vi "main_tweezer_program.vi"() -> ()   [LabVIEW 2017]
uses:
  <vilib>/userdefined/High Color/IMAQdx.ctl
  Serial - Settings.ctl
  <vilib>/Platform/TimedLoop/XDataNode/timing_clust.ctl
  <vilib>/Platform/TimedLoop/XDataNode/nitl_modes.ctl
  <vilib>/Platform/TimedLoop/XDataNode/wakeup.ctl
  C:/Users/mcroning/Documents/builds/Tweezers211_2020/Optical Tweezers Source Tufts/ThorLabs.MotionControl.KCube.PositionAlignerCLI.dll
  ThorLabs.MotionControl.KCube.PositionAlignerCLI.dll
  <vilib>/DAQmx/read.llb/DAQmx Read (Analog DBL 1Chan 1Samp).vi
  <vilib>/DAQmx/write.llb/DAQmx Write (Analog DBL 1Chan 1Samp).vi
  <vilib>/DAQmx/write.llb/DAQmx Write (Analog 1D DBL NChan 1Samp).vi
  <vilib>/DAQmx/read.llb/DAQmx Read (Analog 1D DBL NChan 1Samp).vi
  <vilib>/Analysis/baseanly.llb/Mean (DBL).vi
  <extravilib>/ChannelInstances/Tag-bool/Read With Abort.vi
  <extravilib>/ChannelInstances/Tag-bool/Write With Abort.vi
  <vilib>/DAQmx/create/channels.llb/DAQmx Create Channel (AI-Voltage-Basic).vi
  <vilib>/DAQmx/create/channels.llb/DAQmx Create Channel (AO-Voltage-Basic).vi
  <vilib>/Instr/_visa.llb/VISA Configure Serial Port (Instr).vi
  <vilib>/DAQmx/miscellaneous.llb/DAQmx Fill In Error Info.vi
  <vilib>/Utility/inputDevices.llb/mouseAcquire.vi
  <extravilib>/ChannelInstances/Tag-bool/Instantiate.vi
  <extravilib>/ChannelInstances/Tag-bool/EndpointRead.vi
  <extravilib>/ChannelInstances/Tag-bool/Endpoint.vi
  <vilib>/addons/control/pid/pid.llb/PID (DBL).vi
  <vilib>/platform/TimedLoop/XDataNode/XDataNode.xnode
  <vilib>/vision/driver/NI_Vision_Acquisition_Software.lvlib
  C:/Users/mcroning/Documents/builds/Tweezers211_2020/Optical Tweezers Source Tufts/Thorlabs.MotionControl.Controls.dll
  Thorlabs.MotionControl.Controls.dll
  <extravilib>/ChannelInstances/Tag-bool.lvlib
  <vilib>/addons/control/pid/NI_PID_autopid.lvlib
  <vilib>/Platform/TimedLoop/XDataNode/XDNodeRunTimeDep.lvlib
  <vilib>/Analysis/NI_AALBase.lvlib
  <vilib>/addons/control/pid/NI_PID_pid.lvlib
  C:/Program Files (x86)/National Instruments/LabVIEW 2017/resource/objmgr/imaqdx.rc
panel:
  in  "Period":i64
  out "Mean Temp":dbl
  out "Mean magnitude":dbl
  out "Mean phase":dbl
  in  "Tab Control":T1(tab)
  in  "Exposure time LS":i32=25000
  in  "Frame rate LS":i32=30
  out "Sensor Readout Mode":string
  in  "Number of Images":i32=5
  in  "Exposure time LSwhile run":i32=30000
  out "Bead":cluster{"X":dbl, "Y":dbl}
  out "Score":i32
  in  "Learn Bead for Tracking":bool
  out "Bead Learned":bool
  in  "autotuning parameters":T2={"controller type"=1, "relay cycles"=3, "relay amplitude"=1.0, "control specification"=2, "PV noise level"=0.1} {"PV noise level" format="%.2f"; "control specification" items=["normal", "fast", "slow"]; "relay amplitude" format="%.2f"; "controller type" items=["PID", "PI", "P"]}
  in  "PID gains":T3={"proportional gain (Kc)"=0.398, "integral time (Ti, min)"=0.01577, "derivative time (Td, min)"=0.0} {"derivative time (Td, min)" format="%.3f"; "integral time (Ti, min)" format="%.3f"; "proportional gain (Kc)" format="%.3f"}
  out "Autotuning PID gains out":T3={"proportional gain (Kc)"=1.0, "integral time (Ti, min)"=0.01, "derivative time (Td, min)"=0.0} {"derivative time (Td, min)" format="%.3f"; "integral time (Ti, min)" format="%.3f"; "proportional gain (Kc)" format="%.3f"}
  out "Heater voltage":dbl format="%.2f"
  in  "Temperature \nupdate period ms":i64=10
  in  "autotune? (F)":bool
  in  "Switch control xy":bool=TRUE
  out "output top":dbl format="%.2e"
  in  "top g pos":bool=TRUE
  in  "bottom g pos":bool=TRUE
  in  "PID pos lock":T3={"proportional gain (Kc)"=1.0, "integral time (Ti, min)"=0.01, "derivative time (Td, min)"=0.0} {"derivative time (Td, min)" format="%.3f"; "integral time (Ti, min)" format="%.3f"; "proportional gain (Kc)" format="%.3f"}
  out "Acum nudge x":dbl
  out "Acum nudge y":dbl
  in  "nudge x+":bool
  in  "nudge y+":bool
  in  "nudge x-":bool
  in  "nudge y-":bool
  in  "Nudge x":dbl min=-0.1 max=0.1 step=0.0001
  in  "Nudge y":dbl min=-0.1 max=0.1 step=0.0001
  out "lock in range x":bool
  out "lock in range y":bool
  out "|X Steering Voltage|<1":bool
  out "|Y Steering Voltage|<1":bool
  in  "proportional":dbl=1.0
  in  "integral":dbl
  in  "differential":dbl
  in  "update PID":bool
  out "Sum":dbl
  out "X demand position":dbl
  out "Y demand position":dbl
  out "lock in range x 2":bool
  out "lock in range y 2":bool
  in  "demand signal scale":dbl=0.1
  out "data to write":dbl[][](array[numeric])
  in  "Record Data":bool
  in  "Write to  file":bool
  out "steering voltages":dbl[](array[numeric])
  in  "lock on":bool
  in  "Set Frequency":dbl=1.0
  out "Objective monitor":dbl
  out "Phase":dbl
  out "ResponseMagnitude":dbl
  out "Temp C":dbl
  in  "Temp Setpoint":dbl format="%.2f"
  out "clicks":i32
  out "Image 2":T4(plugin-control)
  in  "stop":bool
  in  "KCubePositionAlignerControl 2":refnum<k24>(container)
  out "Mouse Initialized":bool
  out "Calib pt":i32
  in  "Calibrate Mouse":bool
  in  "Calib scale":dbl=0.1
  in  "Mouse Active":bool
  out "Y":dbl
  out "X":dbl
  in  "Focus Increment":dbl=0.1 min=0.0 max=1.0 step=0.001
  in  "Focus out":dbl min=0.0 max=10.0 step=0.01
  # "Program designed for automatic rheology measurements"
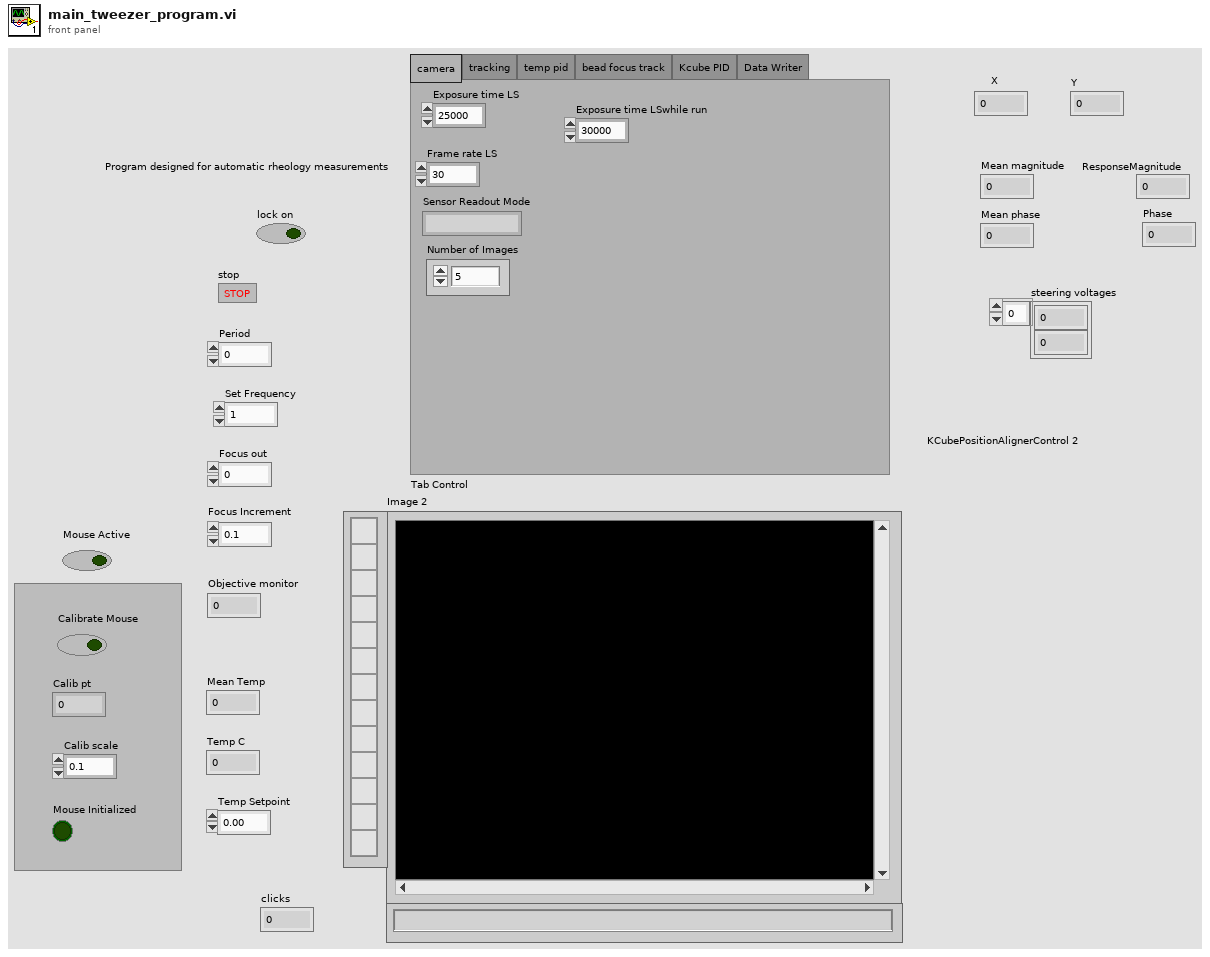
[diagram p1: front panel]
types:
  T1 = enum32{"camera", "tracking", "temp pid", "bead focus track", "Kcube PID", "Data Writer"}
  T2 = cluster{"controller type":u16, "relay cycles":i32, "relay amplitude":dbl, "control specification":u16, "PV noise level":dbl}
  T3 = cluster{"proportional gain (Kc)":dbl, "integral time (Ti, min)":dbl, "derivative time (Td, min)":dbl}
  T4 = typedef "IMAQ Image.ctl" = refnum<image>
  T5 = typedef "Serial - Settings.ctl" = cluster{"baud rate":u32, "data bits":u16, "parity":enum16{"None", "Odd", "Even", "Mark", "Space"}, "stop bits":u16, "flow control":u16}
  T6 = typedef "IMAQdx.ctl" = refnum<k21>
  T7 = typedef "IMAQ Object Tracking Session.ctl" = refnum<k20>
  T8 = cluster{cluster{"Horizontal":i32, "Vertical":i32}, dbl[]}[]
  T9 = cluster{"button 1":bool, "button 2":bool, "button 3":bool, "button 4":bool}
  T10 = cluster{"Horizontal":i32, "Vertical":i32, "Scrolling":i32}
  T11 = cluster{cluster{"Horizontal":i32, "Vertical":i32}, dbl[]}
  T12 = typedef "NI_Matrix.lvlib/RealMatrix.ctl" = dbl[][]
  T13 = cluster{"transformation matrix":T12, "offset":dbl[]}
  T14 = typedef "LVPoint32TypeDef.ctl" = cluster{"Horizontal":i32, "Vertical":i32}
  T15 = cluster{"Global Rectangle":i32[], "Contours":cluster{"Contour Type":u32, "ROI Type":u32, "Points":i32[]}[]}
  T16 = typedef "XDNodeRunTimeDep.lvlib/timing_clust.ctl" = cluster{"Expected End [f-1]":u64, "Actual End [f-1]":u64, "Finished Late? [f-1]":bool, "Expected End [i-1]":u64, "Actual End [i-1]":u64, "Finished Late? [i-1]":bool, "Expected Start [i]":u64, "Actual Start [i]":u64, "Expected Start [f]":u64, "Actual Start [f]":u64, "Source Name":string, "Structure Name":string, "Period":i64, "Deadline":i64, "Offset":i64, "Start":i64, "Priority":i32, "Timeout":i32, "Mode":T17, "Wakeup Reason":T18, "Error":errorcluster, "Source Type":string, "Secondary Source Type":string, "Global End Time":u64, "Global Start Time":u64, "Frame Duration":u64, "Iteration Duration":u64, "Assigned CPU":i32, "I/O Scan Engine Mode":u32}
  T17 = typedef "XDNodeRunTimeDep.lvlib/nitl_modes.ctl" = enum32{"No Change", "Process missed periods, maintain original phase", "Discard missed periods, maintain original phase", "Process missed periods, ignore original phase", "Discard missed periods, ignore original phase"}
  T18 = typedef "XDNodeRunTimeDep.lvlib/wakeup.ctl" = enum32{"Normal", "Aborted", "Asynchronous wakeup", "Timing source error", "Timed loop error", "Timeout"}
  T19 = cluster{"Label":string, "Score":i32, "Angle":dbl, "Location":cluster{"X":dbl, "Y":dbl}, "Bounding Box":cluster{"X":dbl, "Y":dbl}[], "Object Found?":bool}[]
  T20 = cluster{"Label":string, "Score":i32, "Angle":dbl, "Location":cluster{"X":dbl, "Y":dbl}, "Bounding Box":cluster{"X":dbl, "Y":dbl}[], "Object Found?":bool}
  T21 = typedef "Tag-bool.lvlib/))Channel.ctl" = refnum<queue>
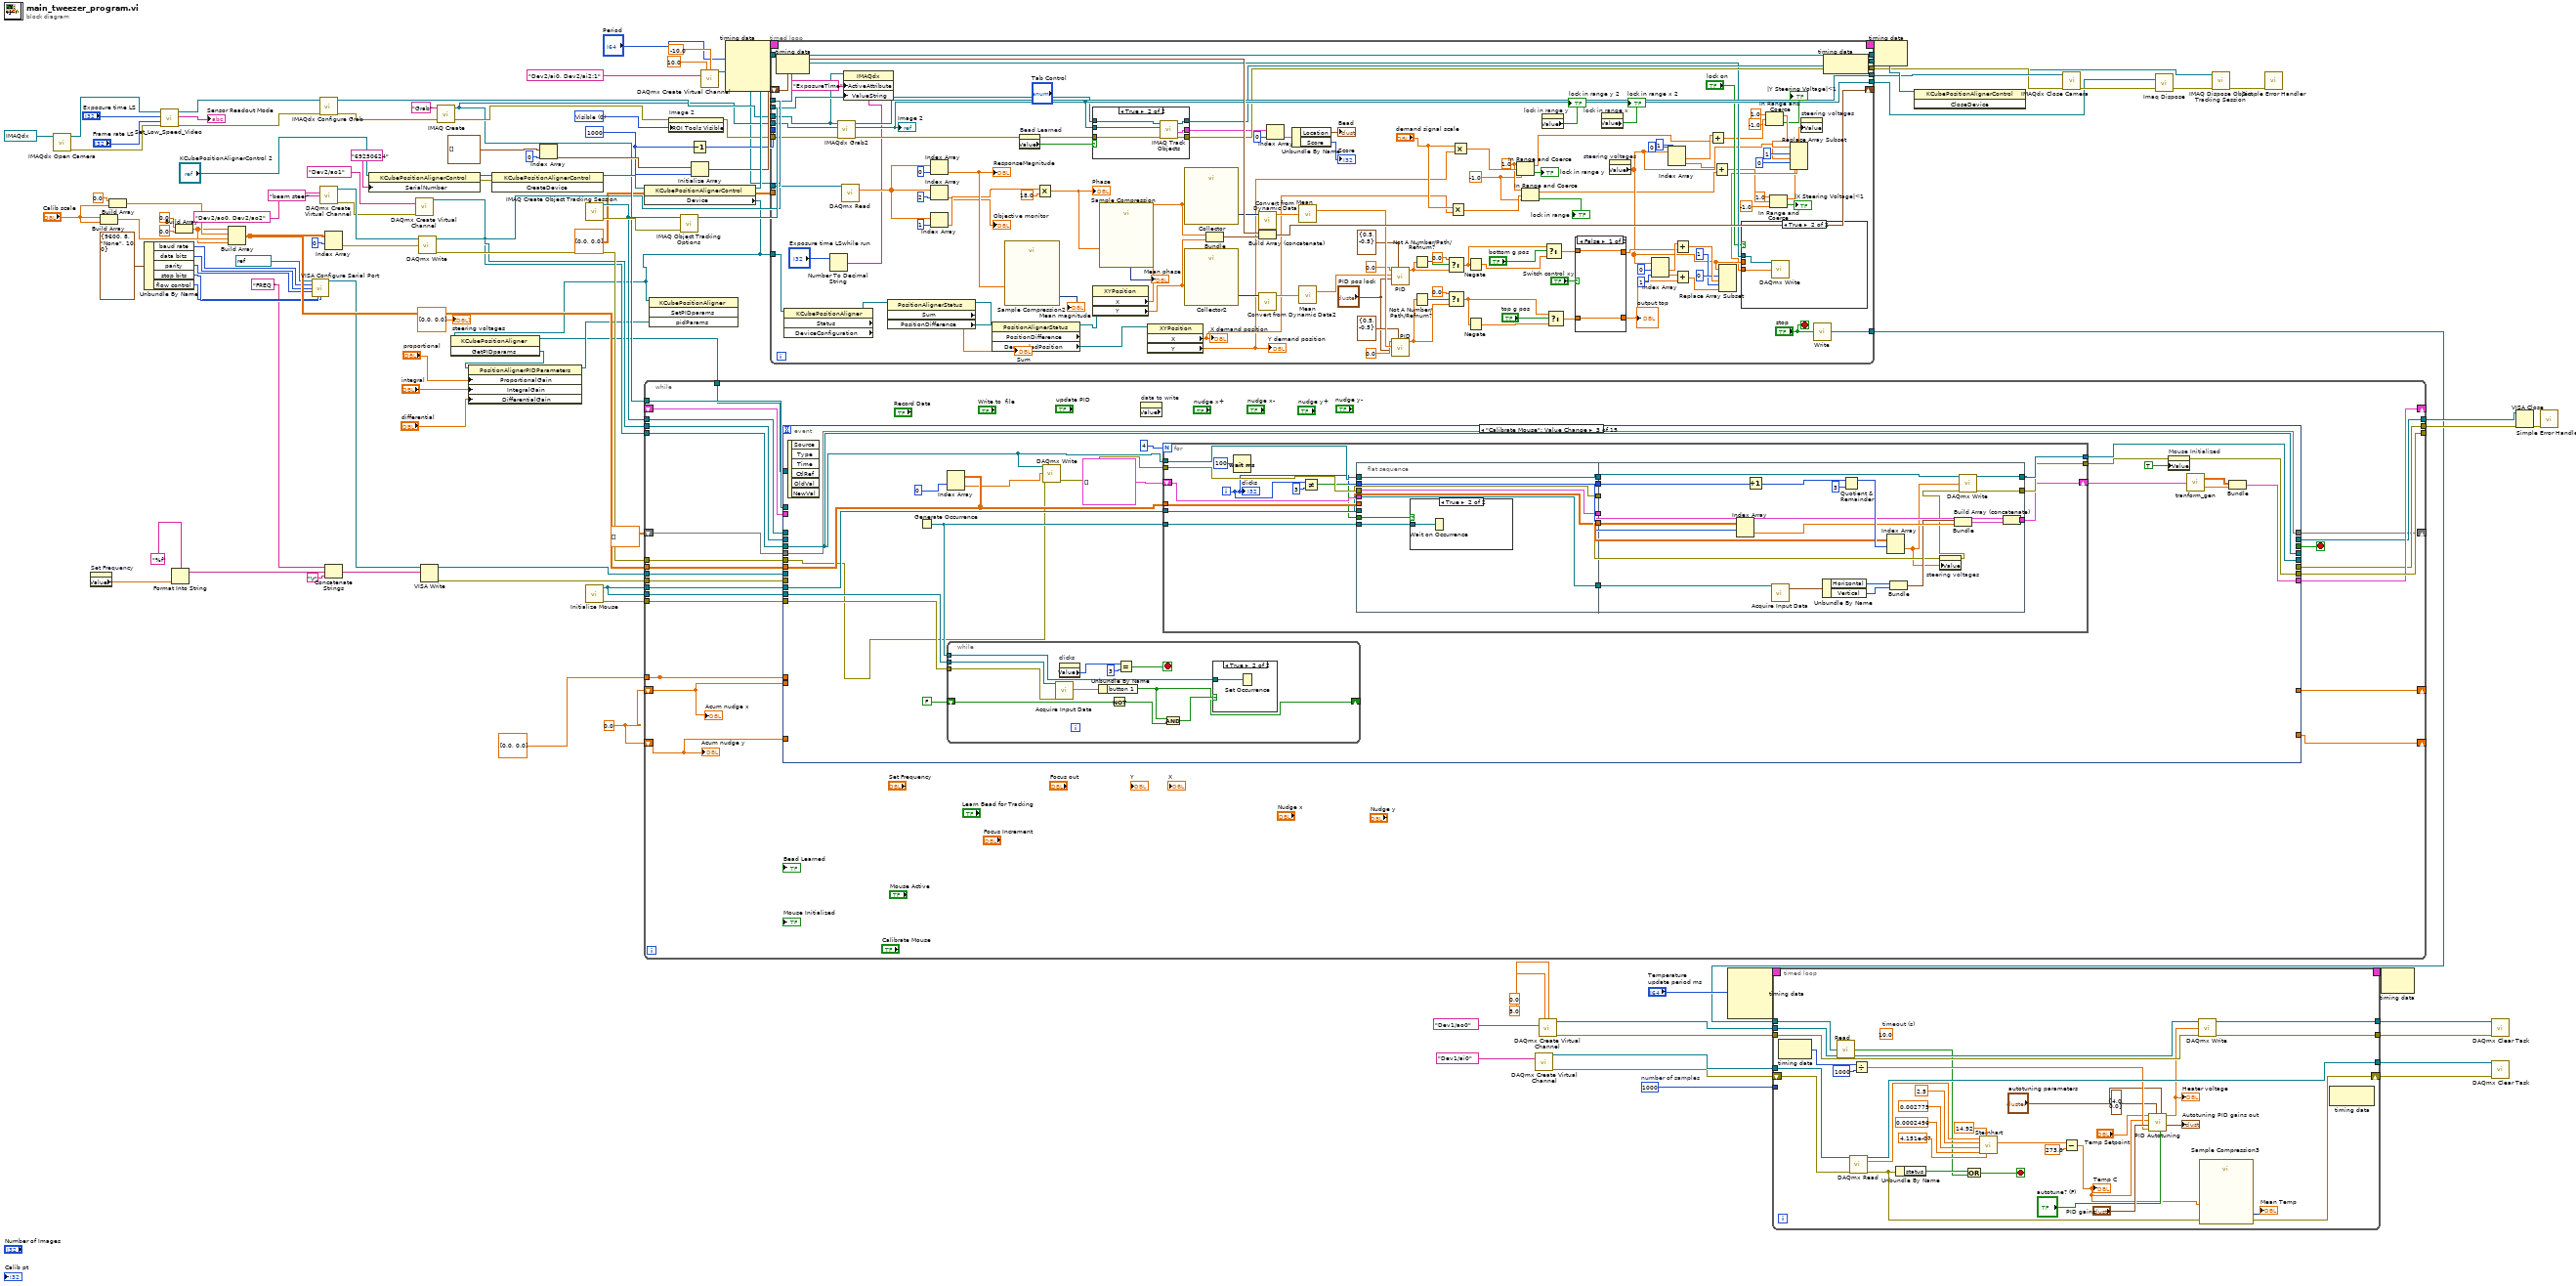
[diagram p0: block diagram]
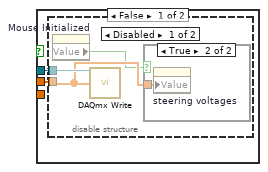
[diagram p3: hidden frame]
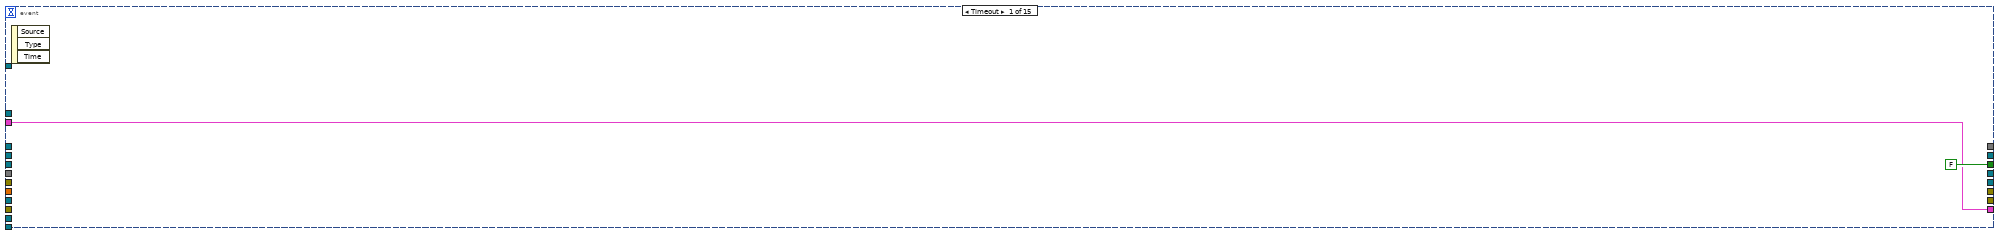
[diagram p7: hidden frame]
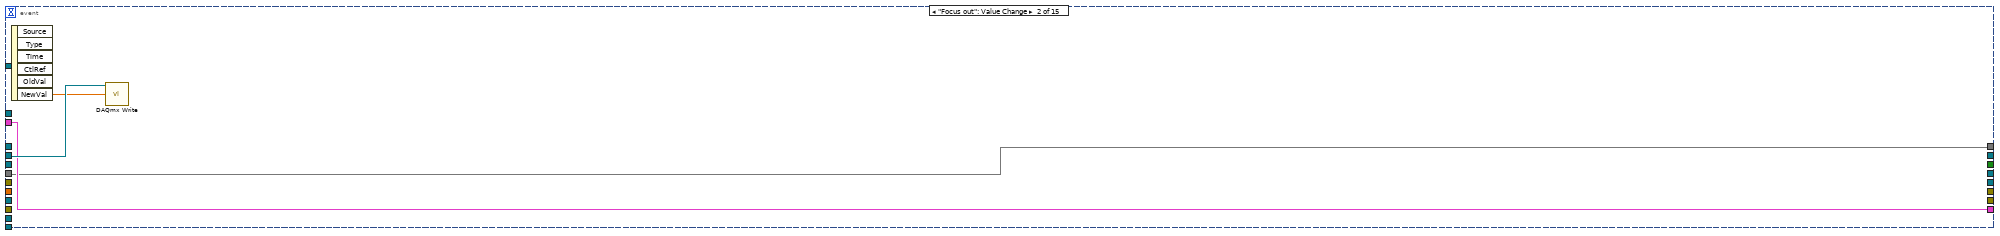
[diagram p8: hidden frame]
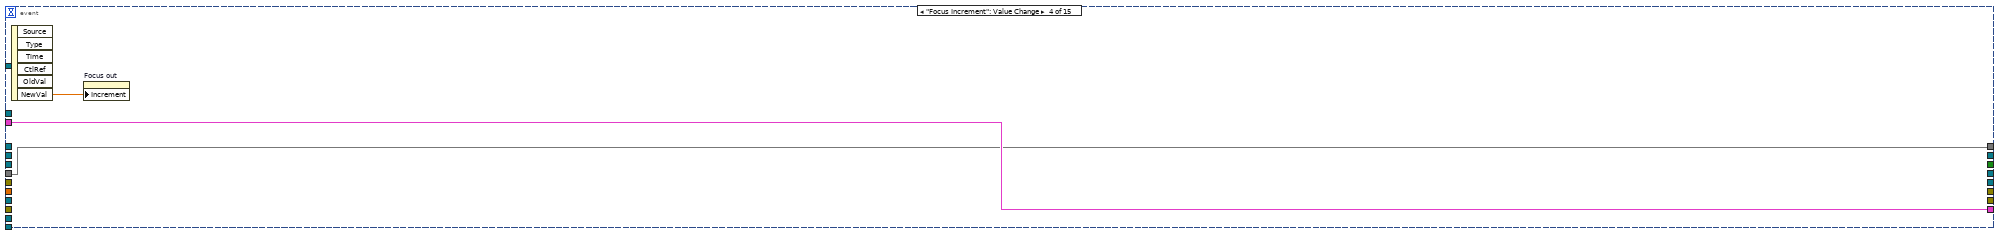
[diagram p11: hidden frame]
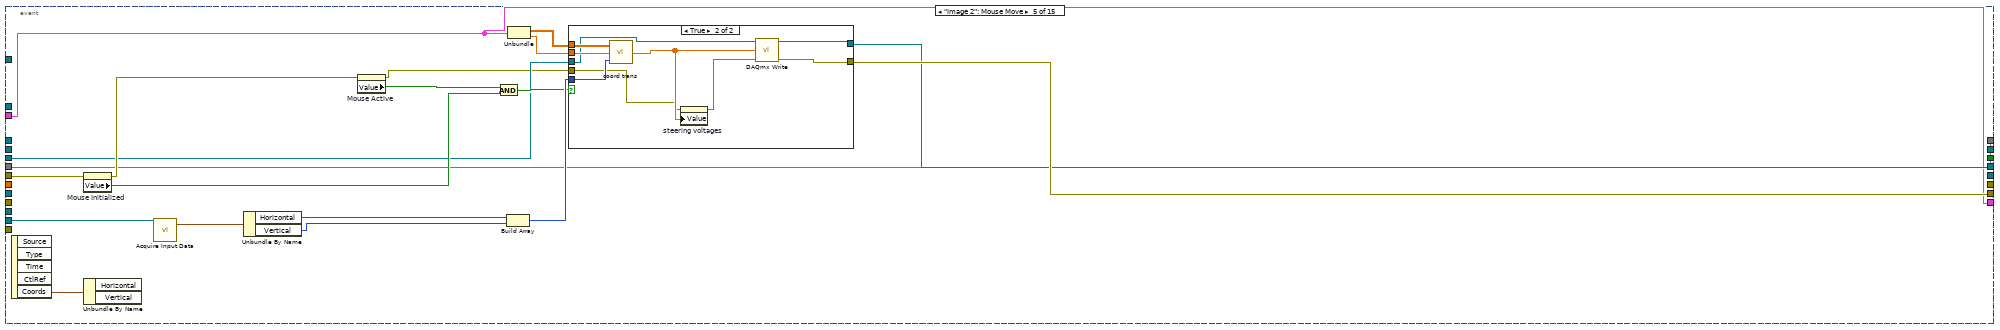
[diagram p12: hidden frame]
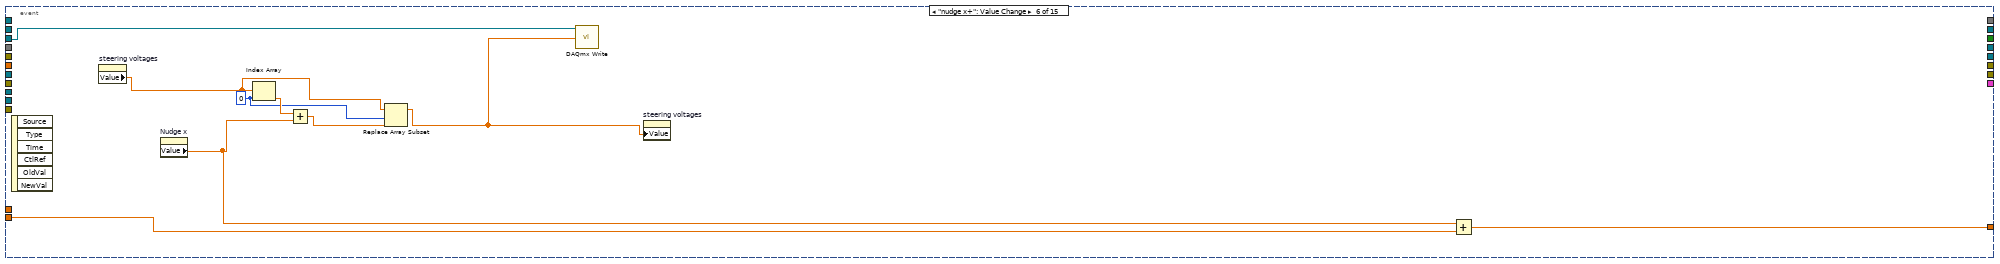
[diagram p14: hidden frame]
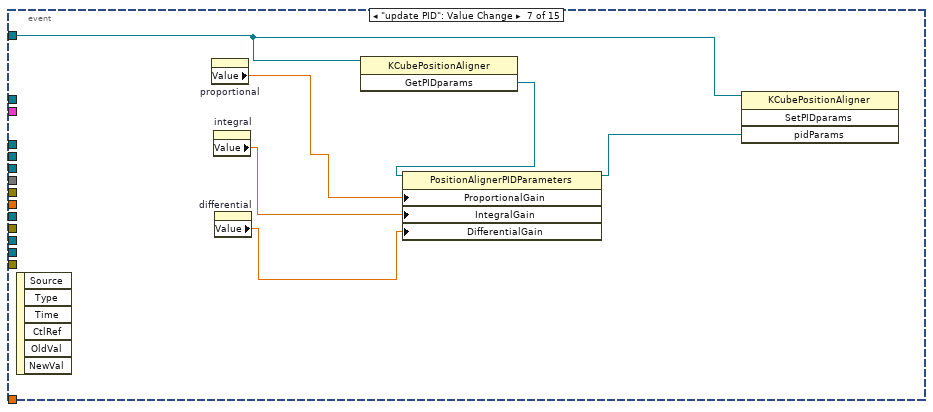
[diagram p15: hidden frame]
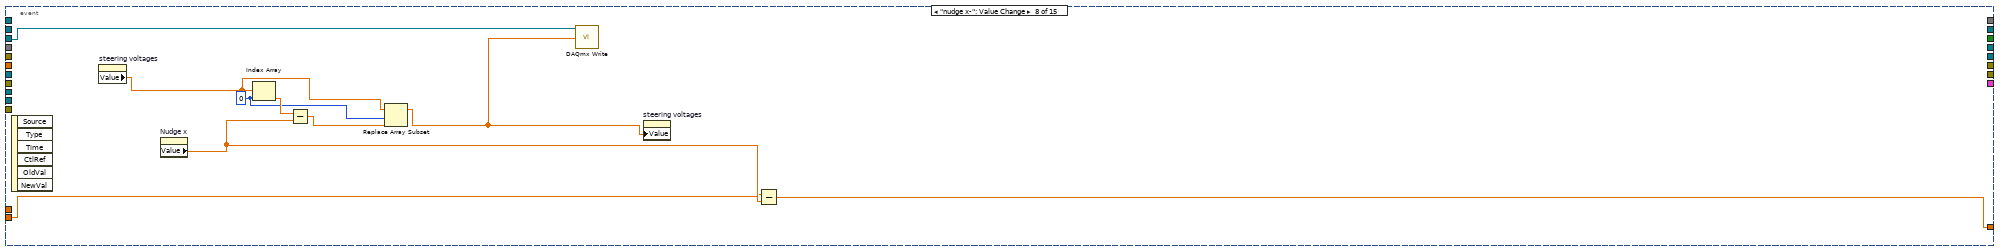
[diagram p16: hidden frame]
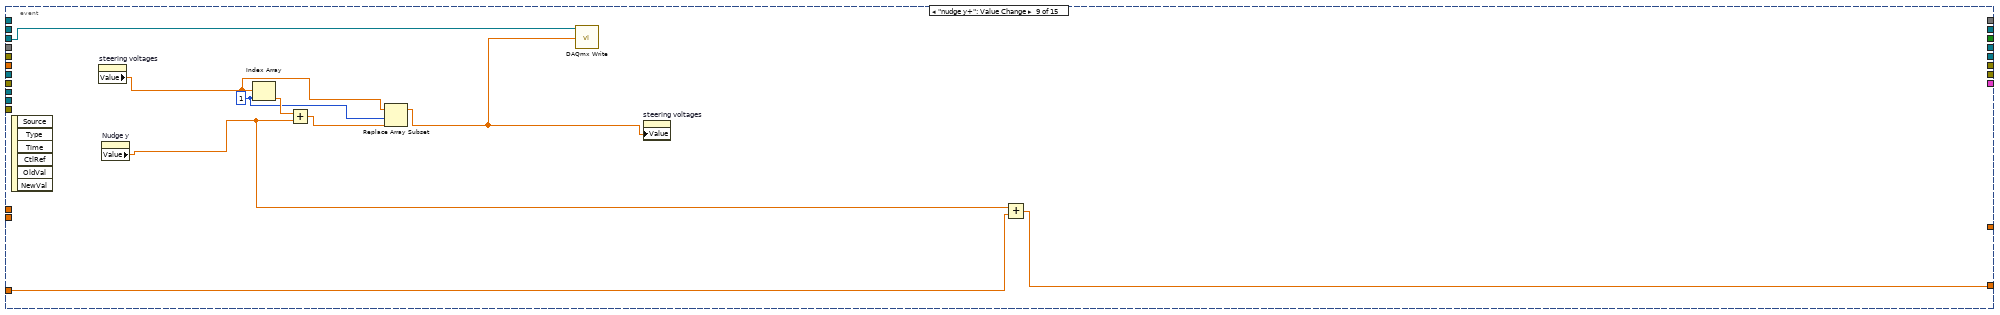
[diagram p17: hidden frame]
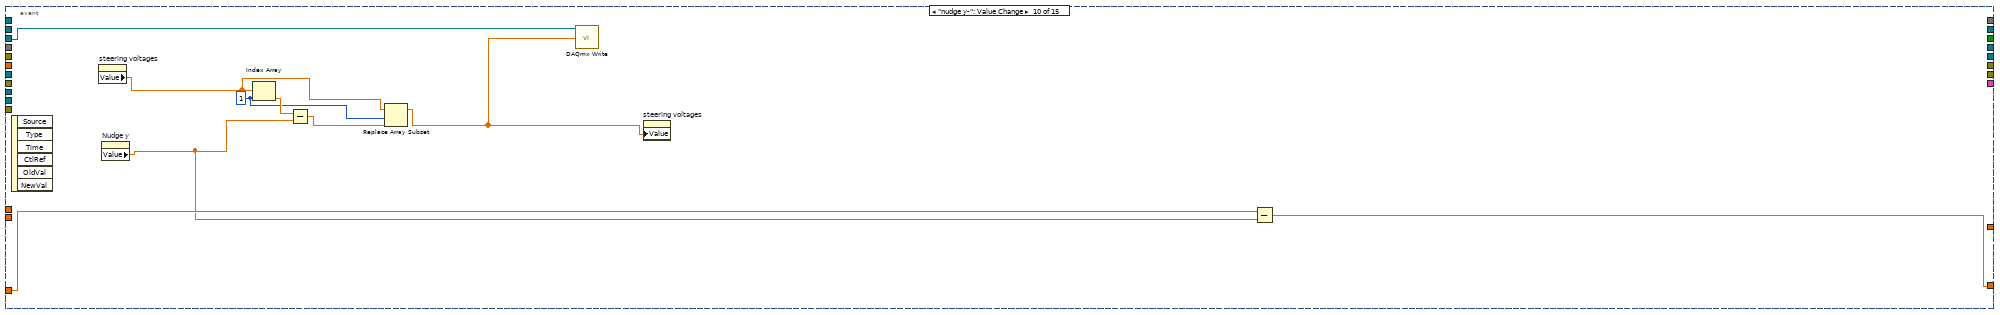
[diagram p18: hidden frame]
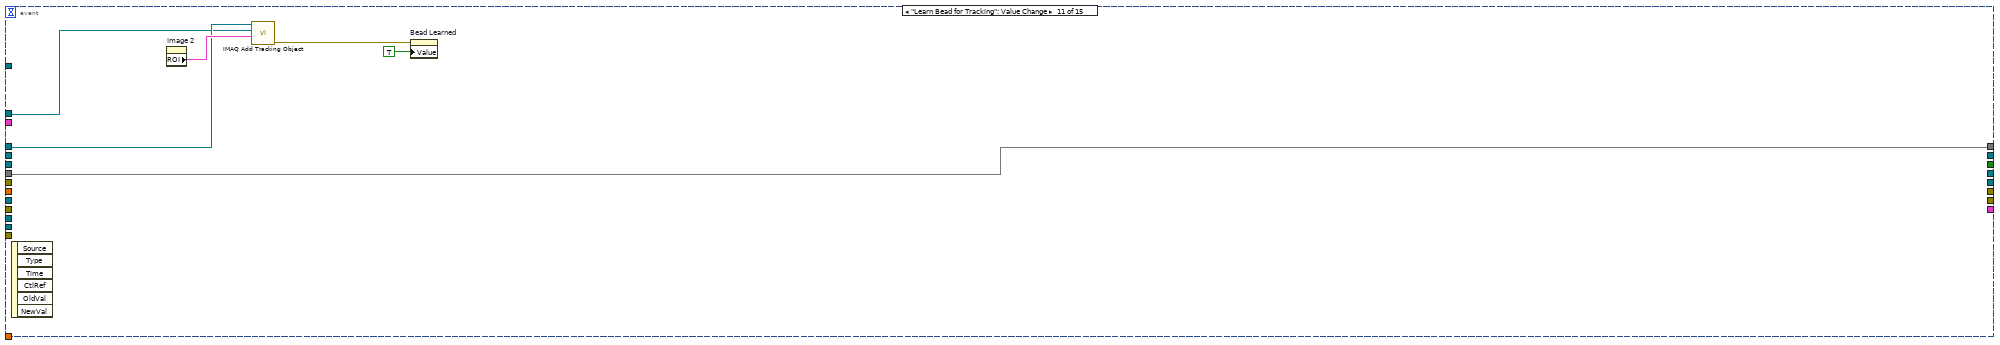
[diagram p19: hidden frame]
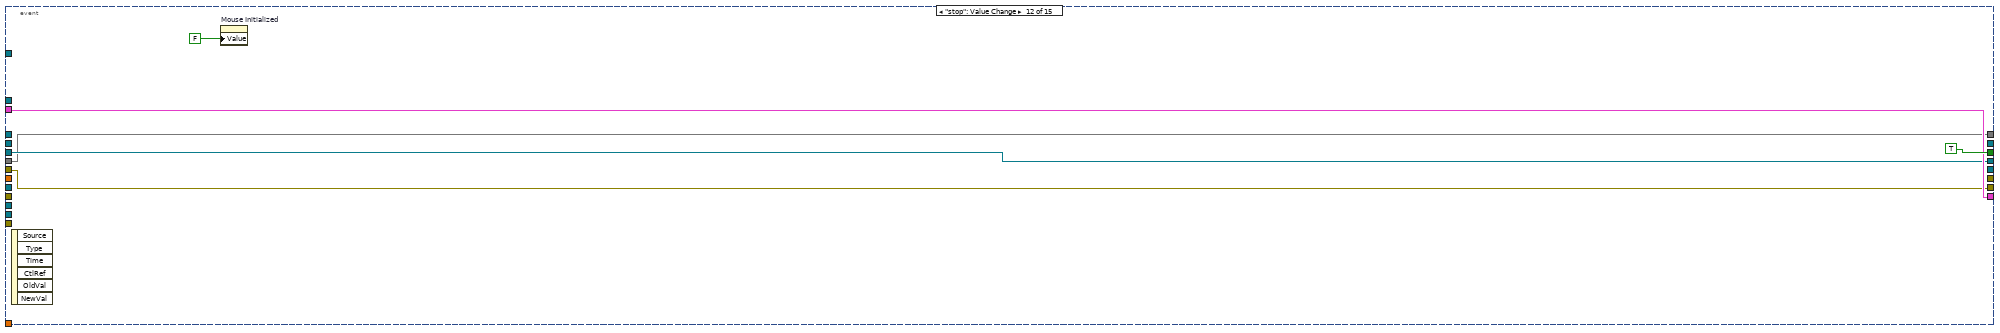
[diagram p20: hidden frame]
diagram:
  w12 = 0.0
  w57 = 1000  # number of samples
  w67 = u32 0 items=["Visible", "Hidden", "Hidden, Use WindTools Palette"] ("ROI Tools Visible")
  w81 = 1000 ("dimension size")
  n1 = call <vilib>:"IMAQdx Open Camera.vi"("Session In"=T6 "cam0") -> ("error out"=w73:errorcluster, "Session Out"=w75:T6)  [unwired: 9 in]
  n2 = property on="Set Frequency" class="DigNum (strict)"() -> ("Value"=w29:dbl)  [unwired: 2 in, 2 out]
  n3 = Build Array("Calib scale", "Calib scale") -> (w107:dbl[])
  n4 = Build Array(0.0 ("element"), "Calib scale") -> (w108:dbl[])
  n5 = Unbundle By Name(T5 {"baud rate"=9600, "data bits"=8, "parity"=enum."None", "stop bits"=10, "flow control"=0} ("Serial Settings")) -> ("baud rate"=w37:u32, "data bits"=w36:u16, "parity"=w35:enum16{"None", "Odd", "Even", "Mark", "Space"}, "stop bits"=w34:u16, "flow control"=w33:u16)
  n6 = call "Set_Low_Speed_Video.vi"("error in (no error)"=w73, "Frame rate LS"="Frame rate LS", "Exposure time LS"="Exposure time LS", "Refnum in"=w75) -> ("error out"=w72:errorcluster, "ValueString"=→"Sensor Readout Mode":string, "Refnum out"=w74:T6)  [unwired: 5 in]
  n7 = Format Into String(format string="%f", w29) -> (resulting string=w30:string)  [unwired: 2 in, 1 out]
  n8 = Build Array(0.0 ("element"), 0.0 ("element")) -> (w102:dbl[])
  n9 = Build Array(w102, w108, w107, w102) -> (w101:dbl[][])
  n10 = call-poly "VISA Configure Serial Port"("VISA resource name"=refnum<visa-resource-name> "COM5", "baud rate (9600)"=w37, "data bits (8)"=w36, "parity (0:none)"=w35, "stop bits (10: 1 bit)"=w34, "flow control (0:none)"=w33) -> ("VISA resource name out"=w28:refnum<visa-resource-name>)  [unwired: 3 in, 6 out]
  n11 = call <vilib>:"IMAQdx Configure Grab.vi"("error in"=w72, "Session In"=w74) -> ("error out"=w89:errorcluster, "Session Out"=w76:T6)  [unwired: 8 in]
  n12 = call-poly <vilib>:"DAQmx Create Virtual Channel.vi"("physical channels"=tag "Dev2/ao0, Dev2/ao2", "name to assign"="beam steer") -> ("task out"=w111:refnum<k21>, "error out"=w14:errorcluster)  [unwired: 12 in]
  n13 = Index Array(array=w101, index (row)=0) -> (element=w105:dbl[])  [unwired: 1 in]
  n14 = Concatenate Strings("FREQ " ("string"), w30, "\r") -> (w26:string)
  n15 = property class="KCubePositionAlignerControl"(reference="KCubePositionAlignerControl 2", "SerialNumber"="69250624" ("SerialNumber 2")) -> (reference out=w97:refnum<k24>, error out=w95:errorcluster)  [unwired: 1 in]
  n16 = call-poly <vilib>:"DAQmx Create Virtual Channel.vi"("physical channels"=tag "Dev2/ao1", "error in"=w14) -> ("task out"=w19:refnum<k21>)  [unwired: 12 in, 1 out]
  n17 = call-poly <vilib>:"DAQmx Write.vi"("task/channels in"=w111, "data"=w105) -> ("task out"=w17:refnum<k21>, "error out"=w100:errorcluster)  [unwired: 11 in, 1 out]
  n18 = VISA Write(VISA resource name=w28, write buffer=w26) -> (VISA resource name out=w27:refnum<visa-resource-name>, error out=w21:errorcluster)  [unwired: 1 in, 1 out]
  n19 = call "IMAQ Create"("Image Name"="Grab", "error in (no error)"=w89) -> ("New Image"=w64:T4, "error out"=w69:errorcluster)  [unwired: 3 in]
  n20 = invoke class="KCubePositionAlignerControl" method="CreateDevice"(reference=w97, error in=w95) -> (reference out=w94:refnum<k24>)  [unwired: 1 in, 2 out]
  n21 = Index Array(array=cluster{"X":dbl, "Y":dbl}[] [], index=0) -> (element=w83:cluster{"X":dbl, "Y":dbl})
  n22 = call "IMAQ Create Object Tracking Session"() -> ("error out"=w66:errorcluster, "Object Tracking Session"=w65:T7)  [unwired: 10 in]
  n23 = call <vilib>:"Initialize Mouse.vi"() -> ("error out"=w71:errorcluster, "device ID"=w70:refnum<k1>)  [unwired: 10 in]
  n24 = property class="KCubePositionAlignerControl"(reference=w94) -> (reference out=w93:refnum<k24>, "Device"=w4:refnum<k24>)  [unwired: 1 in, 1 out]
  n25 = invoke class="KCubePositionAligner" method="GetPIDparams"(reference=w4) -> (reference out=w2:refnum<k24>, "GetPIDparams"=w3:refnum<k24>)  [unwired: 2 in, 1 out]
  n26 = property class="PositionAlignerPIDParameters"(reference=w3, "ProportionalGain"="proportional", "IntegralGain"="integral", "DifferentialGain"="differential") -> (reference out=w8:refnum<k24>)  [unwired: 1 in, 1 out]
  n27 = while {
    tunnel: w19 -> [w137]
    tunnel: w17 -> [w135]
    tunnel: w101 -> [w136]
    tunnel: w100 -> [w134]
    tunnel: [w133] -> _
    shift-right: [w132] -> _
    shift-left: _ -> [w131]
    tunnel: w71 -> [w130]
    tunnel: w70 -> [w129]
    tunnel: w70 -> [w128]
    tunnel: w65 -> [w127]
    tunnel: w64 -> [w126]
    tunnel: w27 -> [w125]
    tunnel: [w124] -> w23
    tunnel: [w123] -> w22
    tunnel: w21 -> [w122]
    shift-right: [w121] -> _
    shift-left: dbl[][] [] -> [w120]
    tunnel: dbl[] [0.0, 0.0] -> [w119]
    tunnel: [w119] -> _
    shift-right: [w118] -> _
    shift-left: w12 -> [w117]
    shift-right: [w115] -> _
    shift-left: w12 -> [w116]
    tunnel: w2 -> [w114]
    stop <- w138 stop-if-true
    n28 = event shown="[2] \"Calibrate Mouse\": Value Change" {
      selector: _ -> [_ _ _ _ _ _ _ _ _ _ _ _ _ _ _]
      dyn-events: _ -> [_ _ _ _ _ _ _ _ _ _ _ _ _ _ _]
      timeout: _ -> [_ _ _ _ _ _ _ _ _ _ _ _ _ _ _]
      tunnel: [FALSE _ _ _ _ _ _ _ _ _ _ TRUE _ _ _] -> w138
      tunnel: w137 -> [_ w144 _ _ _ _ _ _ _ _ _ _ _ _ _]
      tunnel: w136 -> [_ _ w152 _ _ _ _ _ _ _ _ _ _ _ _]
      tunnel: w135 -> [_ _ w146 _ w239 w268 _ w283 w292 w301 _ w309 _ _ _]
      tunnel: [_ _ w146 _ w236 _ _ _ _ _ _ w309 _ _ _] -> _
      tunnel: w134 -> [_ _ w147 _ w244 _ _ _ _ _ _ w310 _ _ _]
      tunnel: [_ _ w164 _ w237 _ _ _ _ _ _ w310 _ _ _] -> w133
      tunnel: [w139 w142 w145 w228 w230 _ _ _ _ _ _ w311 _ _ _] -> w132
      tunnel: w131 -> [w139 w142 _ w228 w230 _ _ _ _ _ _ w311 _ _ _]
      tunnel: w130 -> [_ _ w149 _ _ _ _ _ _ _ _ _ _ _ _]
      tunnel: w129 -> [_ _ w159 _ _ _ _ _ _ _ _ _ _ _ _]
      tunnel: w128 -> [_ _ w158 _ w235 _ _ _ _ _ _ _ _ _ _]
      tunnel: [_ _ w157 _ _ _ _ _ _ _ _ _ _ _ _] -> _
      tunnel: w127 -> [_ _ _ _ _ _ _ _ _ _ w306 _ _ _ _]
      tunnel: w126 -> [_ _ _ _ _ _ _ _ _ _ w305 _ _ _ _]
      tunnel: w125 -> [_ _ _ _ _ _ _ _ _ _ _ _ w320 _ _]
      tunnel: [_ _ _ _ _ _ _ _ _ _ _ _ w317 _ _] -> w124
      tunnel: [_ _ _ _ _ _ _ _ _ _ _ _ w316 _ _] -> w123
      tunnel: w122 -> [_ _ _ _ _ _ _ _ _ _ _ _ w315 _ _]
      tunnel: [_ w141 w153 w227 w231 _ _ _ _ _ w302 w308 w314 w331 w333] -> w121
      tunnel: w120 -> [_ w141 w153 w227 w231 _ _ _ _ _ w302 w308 w314 w329 w334]
      tunnel: w119 -> [_ _ _ _ _ _ _ _ _ _ _ _ _ _ _]
      tunnel: w117 -> [_ _ _ _ _ w262 _ w276 _ _ _ _ _ _ _]
      tunnel: [_ _ _ _ _ w260 _ w275 _ _ _ _ _ _ _] -> w118
      tunnel: w116 -> [_ _ _ _ _ _ _ _ w286 w295 _ _ _ _ _]
      tunnel: [_ _ _ _ _ _ _ _ w284 w293 _ _ _ _ _] -> w115
      tunnel: w114 -> [_ _ _ _ _ _ w270 _ _ _ _ _ _ _ _]
      event Timeout {
        n29 = event-data() -> ()  [unwired: 1 in, 3 out]
      }
      event "Focus out": Value Change {
        n30 = event-data() -> ("NewVal"=w143:dbl)  [unwired: 1 in, 5 out]
        n31 = call-poly <vilib>:"DAQmx Write.vi"("task/channels in"=w144, "data"=w143) -> ()  [unwired: 11 in, 3 out]
      }
      event "Calibrate Mouse": Value Change {
        n32 = event-data() -> ()  [unwired: 1 in, 6 out]
        n33 = Generate Occurrence() -> (w162:refnum<k4>)
        n34 = Index Array(array=w152, index (row)=0) -> (element=w150:dbl[])  [unwired: 1 in]
        n35 = while {
          tunnel: w162 -> [w224]
          shift-right: [w221] -> _
          shift-left: FALSE ("button 1") -> [w223]
          tunnel: w149 -> [w219]
          tunnel: w158 -> [w218]
          stop <- w215 stop-if-true
          n36 = call-poly <vilib>:"Acquire Input Data.vi"("device ID"=w218, "error in (no error)"=w219) -> ("button info"=w225:T9)  [unwired: 14 in, 3 out]
          n37 = property on="clicks" class="DigNum (strict)"() -> ("Value"=w217:i32)  [unwired: 2 in, 2 out]
          n38 = Unbundle By Name(w225) -> ("button 1"=w221:bool)
          n39 = Not(x=w223) -> (.not. x?=w220:bool)
          n40 = Equal?(x=w217, y=3) -> (x = y?=w215:bool)
          n41 = And(x=w221, y=w220) -> (x .and. y?=w222:bool)
          n42 = case shown="True" w222 {
            tunnel: w224 -> [_ w226]
            frame False {
            }
            frame True {
              n43 = Set Occurrence(w226) -> ()
            }
          }
        }
        n44 = call-poly <vilib>:"DAQmx Write.vi"("task/channels in"=w146, "data"=w150, "error in"=w147) -> ("error out"=w148:errorcluster)  [unwired: 10 in, 2 out]
        n45 = for {
          N: 4 -> [_]
          tunnel: w162 -> [w185]
          tunnel: w159 -> [w183]
          tunnel: w146 -> [w180]
          tunnel: w152 -> [w179]
          tunnel: w148 -> [w176]
          tunnel: [w174] -> w157
          tunnel: [w173] -> w156
          shift-right: [w172] -> w155
          shift-left: T8 [] -> [w170]
          i -> [w169]
          n46 = Wait (ms)(milliseconds to wait=u32 100) -> ()  [unwired: 1 out]
          n47 = Not Equal?(x=w169, y=3) -> (x != y?=w167:bool)
          n48 = flat-sequence {
            tunnel: w185 -> [w193]
            tunnel: [w192] -> w184
            tunnel: w183 -> [w192]
            tunnel: [w191] -> w181
            tunnel: w180 -> [w191]
            tunnel: w179 -> [w190]
            tunnel: [w190] -> w178
            tunnel: w169 -> [w189]
            tunnel: [w189] -> w177
            tunnel: w176 -> [w188]
            tunnel: [w188] -> w175
            tunnel: [w187] -> w171
            tunnel: w170 -> [w187]
            tunnel: w167 -> [w186]
            tunnel: w184 -> [w214]
            tunnel: w181 -> [w205]
            tunnel: w178 -> [w204]
            tunnel: w177 -> [w202]
            tunnel: w175 -> [w197]
            tunnel: [w201] -> w174
            tunnel: [w200] -> w173
            tunnel: [w199] -> w172
            tunnel: w171 -> [w198]
            frame #0 {
              n49 = case shown="True" w186 {
                tunnel: w193 -> [_ w194]
                frame False {
                }
                frame True {
                  n50 = Wait on Occurrence(2:w194) -> ()  [unwired: 2 in, 1 out]
                }
              }
            }
            frame #1 {
              n51 = Index Array(array=w204, index (row)=w202) -> (element=w207:dbl[])  [unwired: 1 in]
              n52 = Increment(x=w202) -> (x+1=w208:i32)
              n53 = call-poly <vilib>:"Acquire Input Data.vi"("device ID"=w214) -> ("axis info"=w213:T10)  [unwired: 15 in, 3 out]
              n54 = Unbundle By Name(w213) -> ("Horizontal"=w212:i32, "Vertical"=w211:i32)
              n55 = Quotient & Remainder(x=w208, y=3) -> (x-y*floor(x/y)=w209:i32)  [unwired: 1 out]
              n56 = Index Array(array=w204, index (row)=w209) -> (element=w195:dbl[])  [unwired: 1 in]
              n57 = Bundle("Horizontal"=w212, "Vertical"=w211) -> (w203:cluster{"Horizontal":i32, "Vertical":i32})  [unwired: 1 in]
              n58 = property on="steering voltages" class="Arr (strict)"(error in=w197, "Value"=w195) -> (error out=w196:errorcluster)  [unwired: 1 in, 1 out]
              n59 = Bundle(w203, w207) -> (w206:T11)  [unwired: 1 in]
              n60 = call-poly <vilib>:"DAQmx Write.vi"("task/channels in"=w205, "data"=w195, "error in"=w196) -> ("task out"=w201:refnum<k21>, "error out"=w200:errorcluster)  [unwired: 10 in, 1 out]
              n61 = Build Array (concatenate)(w198, w206) -> (w199:T8)
            }
          }
          "clicks" <- w169
        }
        n62 = property on="Mouse Initialized" class="Bool (strict)"(error in=w156, "Value"=TRUE ("Mouse Initialized")) -> (error out=w164:errorcluster)  [unwired: 1 in, 1 out]
        n63 = call "tranform_gen.vi"("Array"=w155) -> ("transformation matrix"=w166:T12, "offset"=w165:dbl[])
        n64 = Bundle("transformation matrix"=w166, "offset"=w165) -> (w145:T13)  [unwired: 1 in]
      }
      event "Focus Increment": Value Change {
        n65 = event-data() -> ("NewVal"=w229:dbl)  [unwired: 1 in, 5 out]
        n66 = property on="Focus out" class="DigNum (strict)"("Increment"=w229) -> ()  [unwired: 2 in, 2 out]
      }
      event "Image 2": Mouse Move {
        n67 = event-data() -> ("Coords"=w246:T14)  [unwired: 1 in, 4 out]
        n68 = property on="Mouse Initialized" class="Bool (strict)"(error in=w244) -> (error out=w240:errorcluster, "Value"=w243:bool)  [unwired: 1 in, 1 out]
        n69 = Unbundle By Name(w246) -> ()  [unwired: 2 out]
        n70 = call-poly <vilib>:"Acquire Input Data.vi"("device ID"=w235) -> ("axis info"=w234:T10)  [unwired: 15 in, 3 out]
        n71 = Unbundle By Name(w234) -> ("Horizontal"=w233:i32, "Vertical"=w232:i32)
        n72 = property on="Mouse Active" class="Bool (strict)"(error in=w240) -> (error out=w238:errorcluster, "Value"=w242:bool)  [unwired: 1 in, 1 out]
        n73 = And(x=w242, y=w243) -> (x .and. y?=w241:bool)
        n74 = Build Array(w233, w232) -> (w245:i32[])
        n75 = Unbundle(w230) -> ("transformation matrix"=w248:T12, "offset"=w247:dbl[])
        n76 = case shown="True" w241 {
          tunnel: w248 -> [_ w259]
          tunnel: w247 -> [_ w258]
          tunnel: w245 -> [_ w257]
          tunnel: w239 -> [w249 w256]
          tunnel: w238 -> [w250 w252]
          tunnel: [w250 w255] -> w237
          tunnel: [w249 w254] -> w236
          frame False {
          }
          frame True {
            n77 = call "coord trans.vi"("x"=w257, "Offset"=w258, "A"=w259) -> ("dgemv"=w253:dbl[])
            n78 = property on="steering voltages" class="Arr (strict)"(error in=w252, "Value"=w253) -> (error out=w251:errorcluster)  [unwired: 1 in, 1 out]
            n79 = call-poly <vilib>:"DAQmx Write.vi"("task/channels in"=w256, "data"=w253, "error in"=w251) -> ("task out"=w254:refnum<k21>, "error out"=w255:errorcluster)  [unwired: 10 in, 1 out]
          }
        }
      }
      event "nudge x+": Value Change {
        w266 = 0 ("index")
        n80 = event-data() -> ()  [unwired: 1 in, 6 out]
        n81 = property on="steering voltages" class="Arr (strict)"() -> ("Value"=w264:dbl[])  [unwired: 2 in, 2 out]
        n82 = property on="Nudge x" class="DigNum (strict)"() -> ("Value"=w261:dbl)  [unwired: 2 in, 2 out]
        n83 = Index Array(array=w264, index=w266) -> (element=w267:dbl)
        n84 = Add(x=w267, y=w261) -> (x+y=w265:dbl)
        n85 = Replace Array Subset(array=w264, new element=w265, index=w266) -> (w263:dbl[])
        n86 = call-poly <vilib>:"DAQmx Write.vi"("task/channels in"=w268, "data"=w263) -> ()  [unwired: 11 in, 3 out]
        n87 = property on="steering voltages" class="Arr (strict)"("Value"=w263) -> ()  [unwired: 2 in, 2 out]
        n88 = Add(x=w261, y=w262) -> (x+y=w260:dbl)
      }
      event "update PID": Value Change {
        n89 = event-data() -> ()  [unwired: 1 in, 6 out]
        n90 = property on="proportional" class="DigNum (strict)"() -> ("Value"=w271:dbl)  [unwired: 2 in, 2 out]
        n91 = property on="integral" class="DigNum (strict)"() -> ("Value"=w272:dbl)  [unwired: 2 in, 2 out]
        n92 = property on="differential" class="DigNum (strict)"() -> ("Value"=w273:dbl)  [unwired: 2 in, 2 out]
        n93 = invoke class="KCubePositionAligner" method="GetPIDparams"(reference=w270) -> ("GetPIDparams"=w274:refnum<k24>)  [unwired: 2 in, 2 out]
        n94 = property class="PositionAlignerPIDParameters"(reference=w274, "ProportionalGain"=w271, "IntegralGain"=w272, "DifferentialGain"=w273) -> (reference out=w269:refnum<k24>)  [unwired: 1 in, 1 out]
        n95 = invoke class="KCubePositionAligner" method="SetPIDparams"(reference=w270, "pidParams"=w269) -> ()  [unwired: 2 in, 4 out]
      }
      event "nudge x-": Value Change {
        w281 = 0 ("index")
        n96 = event-data() -> ()  [unwired: 1 in, 6 out]
        n97 = property on="steering voltages" class="Arr (strict)"() -> ("Value"=w279:dbl[])  [unwired: 2 in, 2 out]
        n98 = property on="Nudge x" class="DigNum (strict)"() -> ("Value"=w277:dbl)  [unwired: 2 in, 2 out]
        n99 = Index Array(array=w279, index=w281) -> (element=w282:dbl)
        n100 = Subtract(x=w282, y=w277) -> (x-y=w280:dbl)
        n101 = Replace Array Subset(array=w279, new element=w280, index=w281) -> (w278:dbl[])
        n102 = call-poly <vilib>:"DAQmx Write.vi"("task/channels in"=w283, "data"=w278) -> ()  [unwired: 11 in, 3 out]
        n103 = property on="steering voltages" class="Arr (strict)"("Value"=w278) -> ()  [unwired: 2 in, 2 out]
        n104 = Subtract(x=w276, y=w277) -> (x-y=w275:dbl)
      }
      event "nudge y+": Value Change {
        w290 = 1 ("index")
        n105 = event-data() -> ()  [unwired: 1 in, 6 out]
        n106 = property on="steering voltages" class="Arr (strict)"() -> ("Value"=w288:dbl[])  [unwired: 2 in, 2 out]
        n107 = property on="Nudge y" class="DigNum (strict)"() -> ("Value"=w285:dbl)  [unwired: 2 in, 2 out]
        n108 = Index Array(array=w288, index=w290) -> (element=w291:dbl)
        n109 = Add(x=w291, y=w285) -> (x+y=w289:dbl)
        n110 = Replace Array Subset(array=w288, new element=w289, index=w290) -> (w287:dbl[])
        n111 = call-poly <vilib>:"DAQmx Write.vi"("task/channels in"=w292, "data"=w287) -> ()  [unwired: 11 in, 3 out]
        n112 = property on="steering voltages" class="Arr (strict)"("Value"=w287) -> ()  [unwired: 2 in, 2 out]
        n113 = Add(x=w285, y=w286) -> (x+y=w284:dbl)
      }
      event "nudge y-": Value Change {
        w299 = 1 ("index")
        n114 = event-data() -> ()  [unwired: 1 in, 6 out]
        n115 = property on="steering voltages" class="Arr (strict)"() -> ("Value"=w297:dbl[])  [unwired: 2 in, 2 out]
        n116 = property on="Nudge y" class="DigNum (strict)"() -> ("Value"=w294:dbl)  [unwired: 2 in, 2 out]
        n117 = Index Array(array=w297, index=w299) -> (element=w300:dbl)
        n118 = Subtract(x=w300, y=w294) -> (x-y=w298:dbl)
        n119 = Replace Array Subset(array=w297, new element=w298, index=w299) -> (w296:dbl[])
        n120 = call-poly <vilib>:"DAQmx Write.vi"("task/channels in"=w301, "data"=w296) -> ()  [unwired: 11 in, 3 out]
        n121 = property on="steering voltages" class="Arr (strict)"("Value"=w296) -> ()  [unwired: 2 in, 2 out]
        n122 = Subtract(x=w295, y=w294) -> (x-y=w293:dbl)
      }
      event "Learn Bead for Tracking": Value Change {
        n123 = event-data() -> ()  [unwired: 1 in, 6 out]
        n124 = property on="Image 2" class="ImageControl"() -> ("ROI"=w307:T15)  [unwired: 2 in, 2 out]
        n125 = call "IMAQ Add Tracking Object"("ROI Descriptor"=w307, "Image"=w305, "Object Tracking Session In"=w306) -> ("error out"=w304:errorcluster)  [unwired: 6 in, 2 out]
        n126 = property on="Bead Learned" class="Bool (strict)"(error in=w304, "Value"=TRUE ("Bead Learned")) -> ()  [unwired: 1 in, 2 out]
      }
      event "stop": Value Change {
        n127 = event-data() -> ()  [unwired: 1 in, 6 out]
        n128 = property on="Mouse Initialized" class="Bool (strict)"("Value"=FALSE ("Mouse Initialized")) -> ()  [unwired: 2 in, 2 out]
      }
      event "Set Frequency": Value Change {
        n129 = event-data() -> ()  [unwired: 1 in, 6 out]
        n130 = property on="Set Frequency" class="DigNum (strict)"() -> ("Value"=w318:dbl)  [unwired: 2 in, 2 out]
        n131 = Format Into String(format string="%f", w318) -> (resulting string=w322:string)  [unwired: 2 in, 1 out]
        n132 = Concatenate Strings("FREQ " ("string"), w322, "\r") -> (w321:string)
        n133 = VISA Write(VISA resource name=w320, write buffer=w321, error in (no error)=w315) -> (VISA resource name out=w317:refnum<visa-resource-name>, error out=w316:errorcluster)  [unwired: 1 out]
      }
      event "Record Data": Value Change {
        n134 = event-data() -> ()  [unwired: 1 in, 6 out]
        n135 = property on="Mean magnitude" class="DigNum (strict)"() -> ("Value"=w328:dbl)  [unwired: 2 in, 2 out]
        n136 = property on="Mean phase" class="DigNum (strict)"() -> ("Value"=w327:dbl)  [unwired: 2 in, 2 out]
        n137 = property on="Set Frequency" class="DigNum (strict)"() -> ("Value"=w332:dbl)  [unwired: 2 in, 2 out]
        n138 = property on="Objective monitor" class="DigNum (strict)"() -> ("Value"=w325:dbl)  [unwired: 2 in, 2 out]
        n139 = property on="Mean Temp" class="DigNum (strict)"() -> ("Value"=w326:dbl)  [unwired: 2 in, 2 out]
        n140 = Build Array(w332, w328, w327, w326, w325) -> (w330:dbl[])
        n141 = Build Array (concatenate)(w329, w330) -> (w331:dbl[][])
        "data to write" <- w331
      }
      event "Write to  file": Value Change {
        n142 = event-data() -> ()  [unwired: 1 in, 6 out]
        n143 = Transpose 2D Array(2D array=w334) -> (transposed array=w333:dbl[][])
        n144 = call "Convert to Dynamic Data2"("2D Array"=w333) -> ("Dynamic Data Type"=w335:dynamicdata)  [unwired: 3 in]
        n145 = call "Write To Measurement File"("Signals"=w335) -> ()  [unwired: 16 in, 3 out]
      }
    }
    n146 = property on="data to write" class="Arr (strict)" props=["Value"]() -> ()  [unwired: 2 in, 3 out]
    "Acum nudge y" <- w116
    "Acum nudge x" <- w117
  }
  n147 = invoke class="KCubePositionAligner" method="SetPIDparams"(reference=w4, "pidParams"=w8) -> ()  [unwired: 2 in, 4 out]
  n148 = property on="Image 2" class="ImageControl"(error in=w69, "ROI Tools Visible"=w67) -> (error out=w68:errorcluster)  [unwired: 1 in, 1 out]
  n149 = call-poly "IMAQ Object Tracking Options"("error in (no error)"=w66, "Object Tracking Session In"=w65) -> ("Object Tracking Session Out"=w63:T7)  [unwired: 7 in, 2 out]
  n150 = Decrement(x=w81) -> (x-1=w80:i32)
  n151 = Initialize Array(w83, w81) -> (w82:cluster{"X":dbl, "Y":dbl}[])
  n152 = call-poly <vilib>:"DAQmx Create Virtual Channel.vi"("maximum value"=10.0, "minimum value"=-10.0, "physical channels"=tag "Dev2/ai0, Dev2/ai2:1") -> ("task out"=w42:refnum<k21>)  [unwired: 11 in, 1 out]
  n153 = node-c288("Period") -> (w10:T16)  [unwired: 3 in]
  n154 = timed-loop {
    tunnel: w93 -> [w448]
    tunnel: [w448] -> w96
    tunnel: w4 -> [w447]
    tunnel: w76 -> [w373]
    tunnel: w64 -> [w446]
    tunnel: w68 -> [w445]
    tunnel: [w437] -> w88
    tunnel: [w436] -> w87
    tunnel: [w431] -> w86
    shift-right: [w439] -> _
    shift-left: w82 -> [w438]
    tunnel: w80 -> [_]
    tunnel: w63 -> [w435]
    tunnel: [w426] -> w62
    tunnel: w42 -> [w424]
    tunnel: [w418] -> w11
    tunnel: dbl[][] [[0.0], [0.0]] -> [_]
    tunnel: w17 -> [w409]
    timing: w10 -> [_]
    timing-out: [_] -> w9
    stop <- "stop" stop-if-true
    w341 = -1.0 ("lower limit")
    w342 = 1.0 ("upper limit")
    n155 = node-c288() -> ()  [unwired: 1 in, 1 out]
    n156 = property class="KCubePositionAligner" props=["Status", "DeviceConfiguration"](reference=w447) -> ("Status"=w444:refnum<k24>)  [unwired: 1 in, 3 out]
    n157 = Number To Decimal String(number="Exposure time LSwhile run") -> (decimal integer string=w370:string)  [unwired: 1 in]
    n158 = call <vilib>:"IMAQdx Grab2.vi"("error in"=w445, "Image In"=w446, "Session In"=w373) -> ("error out"=w433:errorcluster, "Image Out"=w436:T4, "Session Out"=w437:T6)  [unwired: 5 in, 1 out]
    "Image 2" <- w436
    n159 = call-poly <vilib>:"DAQmx Read.vi"("task/channels in"=w424) -> ("data"=w420:dbl[])  [unwired: 12 in, 2 out]
    n160 = property class="IMAQdx"(reference=w373, "ActiveAttribute"="ExposureTime", "ValueString"=w370) -> ()  [unwired: 1 in, 2 out]
    n161 = property class="PositionAlignerStatus"(reference=w444) -> (reference out=w443:refnum<k24>, "Sum"=→"Sum":dbl, "PositionDifference"=w441:refnum<k24>)  [unwired: 1 in, 1 out]
    n162 = Index Array(array=w420, index=0) -> (element=w377:dbl)
    "ResponseMagnitude" <- w377
    n163 = Index Array(array=w420, index=2) -> (element=→"Objective monitor":dbl)
    n164 = Index Array(array=w420, index=1) -> (element=w369:dbl)
    n165 = property class="PositionAlignerStatus" props=["PositionDifference", "DemandedPosition"](reference=w443) -> ("DemandedPosition"=w367:refnum<k24>)  [unwired: 1 in, 3 out]
    n166 = call "Sample Compression2"("Signals"=w377) -> ("Mean"=→"Mean magnitude":dynamicdata)  [unwired: 8 in, 2 out]
    n167 = property on="Bead Learned" class="Bool (strict)"(error in=w433) -> (error out=w432:errorcluster, "Value"=w434:bool)  [unwired: 1 in, 1 out]
    n168 = Multiply(x=w369, y=18.0) -> (x*y=w375:dbl)
    "Phase" <- w375
    n169 = case shown="True" w434 {
      tunnel: w436 -> [_ w471]
      tunnel: w435 -> [w464 w470]
      tunnel: w432 -> [w465 w469]
      tunnel: [w465 w468] -> w431
      tunnel: [_ w467] -> w430
      tunnel: [w464 w466] -> w426
      frame False {
      }
      frame True {
        n170 = call "IMAQ Track Objects"("error in (no error)"=w469, "Image"=w471, "Object Tracking Session In"=w470) -> ("error out"=w468:errorcluster, "Objects (pixel)"=w467:T19, "Object Tracking Session Out"=w466:T7)  [unwired: 4 in, 2 out]
      }
    }
    n171 = property class="XYPosition"(reference=w441) -> ("X"=w398:dbl, "Y"=w396:dbl)  [unwired: 1 in, 2 out]
    n172 = call "Sample Compression"("Signals"=w375) -> ("Mean"=→"Mean phase":dynamicdata)  [unwired: 8 in, 2 out]
    n173 = property class="XYPosition"(reference=w367) -> ("X"=w360:dbl, "Y"=w359:dbl)  [unwired: 1 in, 2 out]
    "X demand position" <- w360
    "Y demand position" <- w359
    n174 = call "Collector"("Signals"=w398) -> ("Collected Signals"=w397:dynamicdata)  [unwired: 9 in, 1 out]
    n175 = call "Collector2"("Signals"=w396) -> ("Collected Signals"=w395:dynamicdata)  [unwired: 9 in, 1 out]
    n176 = Bundle("X"=w398, "Y"=w396) -> (w440:cluster{"X":dbl, "Y":dbl})  [unwired: 1 in]
    n177 = Build Array (concatenate)(w438, w440) -> (w439:cluster{"X":dbl, "Y":dbl}[])
    n178 = call "Convert from Dynamic Data"("Dynamic Data Type"=w397) -> ("Array"=w417:dbl[])  [unwired: 3 in]
    n179 = call "Convert from Dynamic Data2"("Dynamic Data Type"=w395) -> ("Array"=w416:dbl[])  [unwired: 3 in]
    n180 = Index Array(array=w430, index=0) -> (element=w428:T20)
    n181 = Unbundle By Name(w428) -> ("Location"=→"Bead":cluster{"X":dbl, "Y":dbl}, "Score"=→"Score":i32)
    n182 = call-poly <vilib>:"Mean.vi"("X"=w417) -> ("mean"=w415:dbl)  [unwired: 1 out]
    n183 = call-poly <vilib>:"Mean.vi"("X"=w416) -> ("mean"=w412:dbl)  [unwired: 1 out]
    n184 = call-poly <vilib>:"PID.vi"("output range"=cluster{"output high":dbl, "output low":dbl} {"output high"=0.5, "output low"=-0.5}, "PID gains"="PID pos lock", "process variable"=w412, "setpoint"=0.0) -> ("output"=w393:dbl)  [unwired: 6 in, 1 out]
    n185 = call-poly <vilib>:"PID.vi"("output range"=cluster{"output high":dbl, "output low":dbl} {"output high"=0.5, "output low"=-0.5}, "PID gains"="PID pos lock", "process variable"=w415, "setpoint"=0.0) -> ("output"=w400:dbl)  [unwired: 6 in, 1 out]
    n186 = Not A Number/Path/Refnum?(number/path/refnum=w393) -> (NaN/Path/Refnum?=w394:bool)
    n187 = Not A Number/Path/Refnum?(number/path/refnum=w400) -> (NaN/Path/Refnum?=w401:bool)
    n188 = Select(t=0.0, s=w394, f=w393) -> (s? t:f=w388:dbl)
    n189 = Select(t=0.0, s=w401, f=w400) -> (s? t:f=w386:dbl)
    n190 = Multiply(x="demand signal scale", y=w360) -> (x*y=w343:dbl)
    n191 = Multiply(x="demand signal scale", y=w359) -> (x*y=w345:dbl)
    n192 = Negate(x=w388) -> (-x=w387:dbl)
    n193 = Negate(x=w386) -> (-x=w385:dbl)
    n194 = In Range and Coerce(upper limit=w342, x=w345, lower limit=w341) -> (coerced(x)=w344:dbl, In Range?=→"lock in range y":bool)
    n195 = In Range and Coerce(upper limit=w342, x=w343, lower limit=w341) -> (coerced(x)=w340:dbl, In Range?=→"lock in range x":bool)
    n196 = property on="lock in range y" class="Bool (strict)"() -> ("Value"=→"lock in range y 2":bool)  [unwired: 2 in, 2 out]
    n197 = Select(t=w388, s="bottom g pos", f=w387) -> (s? t:f=w382:dbl)
    n198 = Select(t=w386, s="top g pos", f=w385) -> (s? t:f=w381:dbl)
    n199 = case shown="False" "Switch control xy" {
      tunnel: w382 -> [w453 w455]
      tunnel: [w452 w455] -> w379
      tunnel: w381 -> [w452 w454]
      tunnel: [w453 w454] -> w380
      frame False {
      }
      frame True {
      }
    }
    "output top" <- w379
    n200 = property on="lock in range x" class="Bool (strict)"() -> ("Value"=→"lock in range x 2":bool)  [unwired: 2 in, 2 out]
    n201 = property on="steering voltages" class="Arr (strict)"() -> ("Value"=w362:dbl[])  [unwired: 2 in, 2 out]
    n202 = Index Array(array=w362, index #1=0 ("index"), index #2=1 ("index")) -> (element #1=w391:dbl, element #2=w390:dbl)
    n203 = Index Array(array=w362, index #1=1 ("index"), index #2=0 ("index")) -> (element #1=w358:dbl, element #2=w357:dbl)
    n204 = Add(x=w391, y=w380) -> (x+y=w405:dbl)
    n205 = Add(x=w390, y=w379) -> (x+y=w402:dbl)
    n206 = Add(x=w358, y=w344) -> (x+y=w355:dbl)
    n207 = Add(x=w357, y=w340) -> (x+y=w351:dbl)
    n208 = Replace Array Subset(array=w362, new element #1=w405, index #1=0 ("index"), new element #2=w402, index #2=1 ("index")) -> ()  [unwired: 1 out]
    n209 = In Range and Coerce(upper limit=1.0, x=w355, lower limit=-1.0) -> (coerced(x)=w354:dbl, In Range?=→"|Y Steering Voltage|<1":bool)
    n210 = In Range and Coerce(upper limit=1.0, x=w351, lower limit=-1.0) -> (coerced(x)=w348:dbl, In Range?=→"|X Steering Voltage|<1":bool)
    n211 = Replace Array Subset(array=w362, new element #1=w354, index #1=1 ("index"), new element #2=w348, index #2=0 ("index")) -> (w356:dbl[])
    n212 = case shown="True" "lock on" {
      tunnel: w409 -> [w457 w463]
      tunnel: w356 -> [_ w462]
      tunnel: w362 -> [w456 _]
      frame False {
        n213 = disable-structure shown="Disabled" {
          disable-tunnel: w457 -> [w460 _]
          disable-tunnel: w456 -> [w459 _]
          frame Disabled {
            n214 = property on="Mouse Initialized" class="Bool (strict)"() -> ("Value"=w458:bool)  [unwired: 2 in, 2 out]
            n215 = call-poly <vilib>:"DAQmx Write.vi"("task/channels in"=w460, "data"=w459) -> ()  [unwired: 11 in, 3 out]
            n216 = case shown="True" w458 {
              tunnel: w459 -> [_ w461]
              frame False {
              }
              frame True {
                n217 = property on="steering voltages" class="Arr (strict)"("Value"=w461) -> ()  [unwired: 2 in, 2 out]
              }
            }
          }
          frame Enabled {
          }
        }
      }
      frame True {
        n218 = call-poly <vilib>:"DAQmx Write.vi"("task/channels in"=w463, "data"=w462) -> ()  [unwired: 11 in, 3 out]
      }
    }
    n219 = property on="steering voltages" class="Arr (strict)"("Value"=w356) -> ()  [unwired: 2 in, 2 out]
    n220 = call <extravilib>:"Write.vi"("element"="stop") -> ("channel"=w418:T21)  [unwired: 1 out]
    n221 = node-c288() -> ()  [unwired: 1 in, 1 out]
  }
  n222 = call-poly <vilib>:"DAQmx Create Virtual Channel.vi"("physical channels"=tag "Dev1/ai0") -> ("task out"=w46:refnum<k21>, "error out"=w45:errorcluster)  [unwired: 13 in]
  n223 = call-poly <vilib>:"DAQmx Create Virtual Channel.vi"("maximum value"=5.0, "minimum value"=0.0, "physical channels"=tag "Dev1/ao0") -> ("task out"=w52:refnum<k21>, "error out"=w50:errorcluster)  [unwired: 11 in]
  n224 = node-c288("Temperature \nupdate period ms") -> (w59:T16)  [unwired: 3 in]
  n225 = timed-loop {
    tunnel: w46 -> [w501]
    tunnel: w57 -> [_]
    tunnel: [w500] -> w55
    shift-right: [w498] -> w56
    shift-left: w45 -> [w499]
    tunnel: w52 -> [w489]
    tunnel: [w488] -> w51
    tunnel: w50 -> [w487]
    tunnel: [w486] -> w49
    timing: w59 -> [_]
    timing-out: [_] -> w58
    tunnel: w11 -> [w474]
    stop <- w502 stop-if-true
    (unwired) 10.0  # timeout (s)
    n226 = node-c288() -> (w485:i64)  [unwired: 1 in]
    n227 = call <extravilib>:"Read.vi"("channel"=w474) -> ("element"=w475:bool)  [unwired: 1 in, 1 out]
    n228 = call-poly <vilib>:"DAQmx Read.vi"("task/channels in"=w501, "error in"=w499) -> ("task out"=w500:refnum<k21>, "data"=w497:dbl, "error out"=w498:errorcluster)  [unwired: 11 in]
    n229 = Divide(x=w485, y=i64 1000) -> (x/y=w482:dbl)
    n230 = Unbundle By Name(w498) -> ("status"=w503:bool)
    n231 = Or(x=w503, y=w475) -> (x .or. y?=w502:bool)
    n232 = call "Steinhart.vi"("c"=4.151e-07, "R1"=14.92, "b"=0.0002496, "a"=0.002775, "Vex"=2.5, "Vm"=w497) -> ("output variable"=w492:dbl)  [unwired: 5 in]
    n233 = Subtract(x=w492, y=273.0) -> (x-y=w473:dbl)
    "Temp C" <- w473
    n234 = call <vilib>:"PID Autotuning.vi"("autotune? (F)"="autotune? (F)", "autotuning parameters"="autotuning parameters", "output range"=cluster{"output high":dbl, "output low":dbl} {"output high"=4.0, "output low"=0.0}, "dt (s)"=w482, "PID gains"="PID gains", "process variable"=w473, "setpoint"="Temp Setpoint") -> ("PID gains out"=→"Autotuning PID gains out":T3, "output"=w478:dbl)  [unwired: 1 in, 2 out]
    "Heater voltage" <- w478
    n235 = call-poly <vilib>:"DAQmx Write.vi"("task/channels in"=w489, "data"=w478, "error in"=w487) -> ("task out"=w488:refnum<k21>, "error out"=w486:errorcluster)  [unwired: 10 in, 1 out]
    n236 = call "Sample Compression3"("Signals"=w473) -> ("Mean"=→"Mean Temp":dynamicdata)  [unwired: 8 in, 2 out]
    n237 = node-c288() -> ()  [unwired: 1 in, 1 out]
  }
  n238 = node-c288(w9) -> ()  [unwired: 1 out]
  n239 = invoke class="KCubePositionAlignerControl" method="CloseDevice"(reference=w96) -> ()  [unwired: 2 in, 3 out]
  n240 = call <vilib>:"IMAQdx Close Camera.vi"("error in"=w86, "Session In"=w88) -> ("error out"=w92:errorcluster)  [unwired: 9 in]
  n241 = call "Imaq Dispose"("Image"=w87, "error in (no error)"=w92) -> ("error out"=w61:errorcluster)  [unwired: 4 in]
  n242 = call "IMAQ Dispose Object Tracking Session"("error in (no error)"=w61, "Object Tracking Session"=w62) -> ("error out"=w60:errorcluster)  [unwired: 9 in]
  n243 = call <vilib>:"Simple Error Handler.vi"("error in (no error)"=w60) -> ()  [unwired: 4 in, 5 out]
  n244 = node-c288(w58) -> ()  [unwired: 1 out]
  n245 = call <vilib>:"DAQmx Clear Task.vi"("task in"=w51, "error in"=w49) -> ()  [unwired: 13 in, 1 out]
  n246 = call <vilib>:"DAQmx Clear Task.vi"("task in"=w55, "error in"=w56) -> ()  [unwired: 13 in, 1 out]
  n247 = VISA Close(VISA resource name=w23, error in (no error)=w22) -> (error out=w24:errorcluster)
  n248 = call <vilib>:"Simple Error Handler.vi"("error in (no error)"=w24) -> ()  [unwired: 1 in, 8 out]
  "steering voltages" <- dbl[] [0.0, 0.0] ("dgemv")
